vi "Connect.vi"(8 "error in":errorcluster, 11 "Serial in":refnum<class "Serial.lvclass">) -> (0 "error out":errorcluster, 3 "Serial out":refnum<class "Serial.lvclass">)   [LabVIEW 2021, in "Serial.lvclass"]
uses:
  Serial.lvclass
  controls/INI FGV States.ctl
  Serial.lvclass/Serial.ctl
  <vilib>/Instr/_visa.llb/VISA Configure Serial Port (Instr).vi
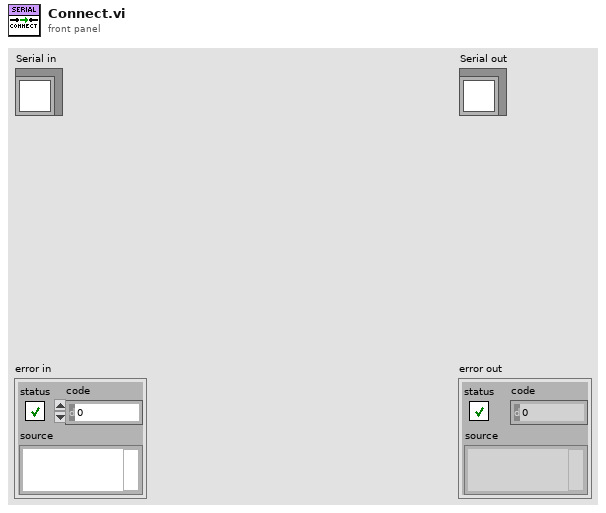
[diagram p1: front panel]
types:
  T1 = typedef "INI FGV States.ctl" = enum16{"Open File", "Read Config", "Write Config", "Close File"}
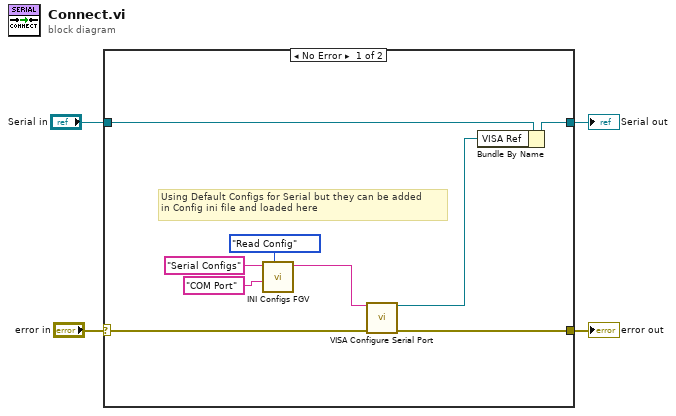
[diagram p0: block diagram]
diagram:
  n1 = case shown="No Error" "error in" {
    selector: "error in" -> [w12 w15]
    tunnel: [w11 w15] -> w3
    tunnel: "Serial in" -> [w13 w14]
    tunnel: [w6 w14] -> w1
    frame No Error {
      # "Using Default Configs for Serial but they can be added\nin Config ini file and loaded here"
      n2 = call "INI Configs FGV.vi"("State"=INI_FGV_States."Read Config", "key"="COM Port", "section"="Serial Configs") -> ("value"=w7:string)  [unwired: 7 in, 1 out]
      n3 = call-poly "VISA Configure Serial Port"("VISA resource name"=w7, "error in (no error)"=w12) -> ("VISA resource name out"=w5:refnum<visa-resource-name>, "error out"=w11:errorcluster)  [unwired: 12 in]
      n4 = Bundle By Name(cluster=w13, "VISA Ref"=w5) -> (w6:refnum<class "Serial.lvclass">)
    }
    frame Error {
    }
  }
  "error out" <- w3
  "Serial out" <- w1
